vi "Waveforms.vi"(8 "Digital Data":digitaldata={"transitions"=[2, 5, 7, 9, 11, 15], "data"=[[1, 0, 1, 0, 1, 0, 1, 0, 1, 0, 1, 1], [0, 1, 0, 1, 1, 0, 1, 0, 0, 0, 0, 0], [1, 0, 0, 1, 1, 0, 0, 1, 0, 1, 1, 0], [0, 0, 1, 0, 0, 1, 0, 0, 1, 0, 0, 0], [1, 0, 0, 1, 0, 0, 1, 0, 1, 0, 1, 0], [1, 1, 0, 0, 1, 1, 0, 1, 1, 0, 0, 1]]}, 9 "Digital Waveform":digitalwaveform(waveform)={"t0"=timestamp(3352482098.6289887 s since 1904-01-01), "dt"=6.0, "Y"={"transitions"=[3, 4, 7], "data"=[[0, 1, 1, 0, 1, 0, 1], [0, 1, 1, 0, 1, 0, 0], [0, 1, 0, 1, 0, 1, 1]]}}, 10 "Waveform 2":waveform(i64)={"t0"=timestamp(3352482085.4272337 s since 1904-01-01), "dt"=8.0, "Y"=[23, 54, 343]}, 11 "Waveform":waveform(dbl)={"t0"=timestamp(3352482079.508895 s since 1904-01-01), "dt"=3.0, "Y"=[11.0, 22.0, 33.0, 44.0]}) -> (3 "All Default Values Are Equal":bool)   [LabVIEW 2010]
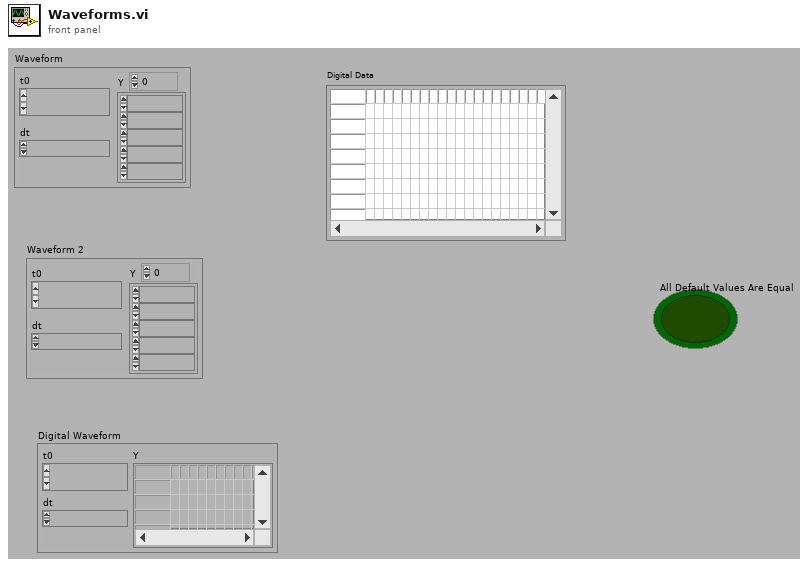
[diagram p1: front panel]
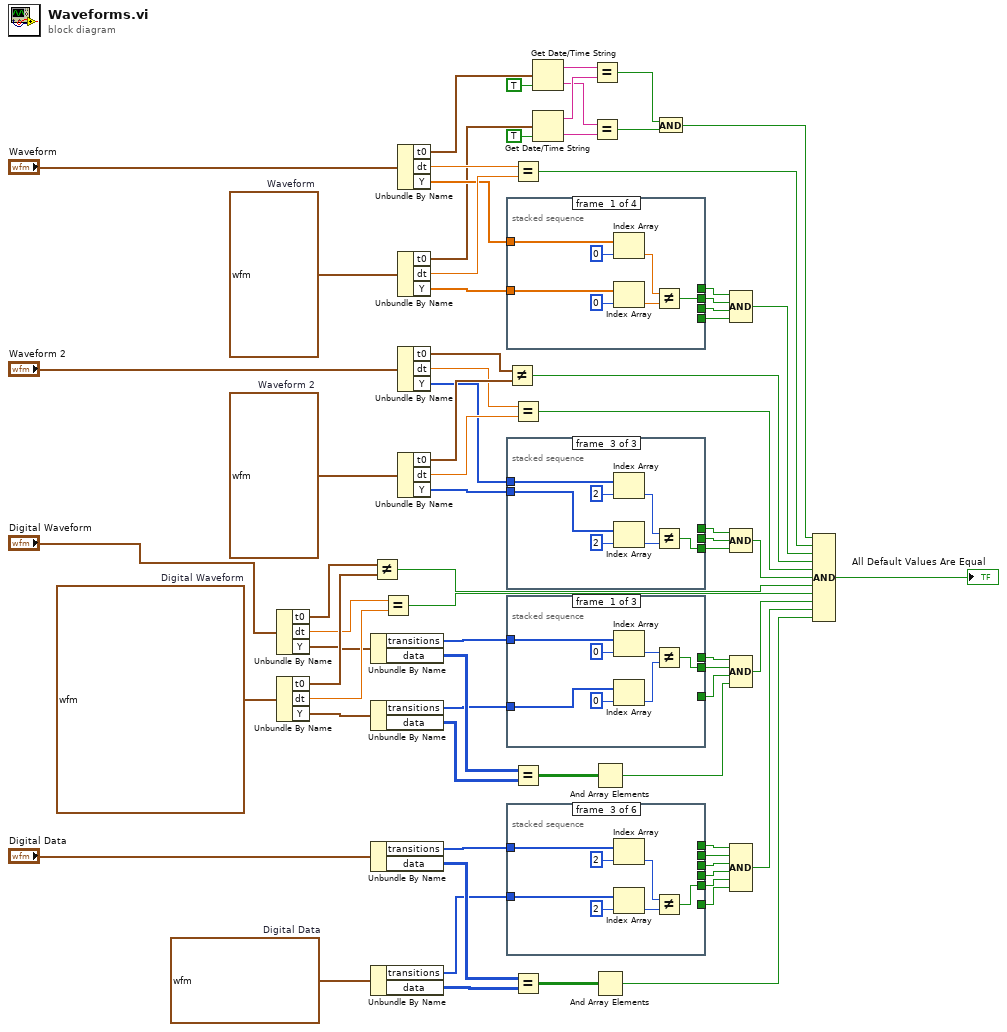
[diagram p0: block diagram]
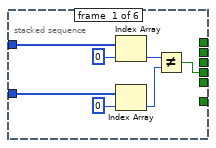
[diagram p2: hidden frame]
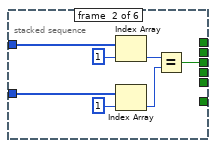
[diagram p3: hidden frame]
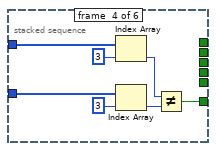
[diagram p4: hidden frame]
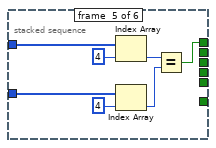
[diagram p5: hidden frame]
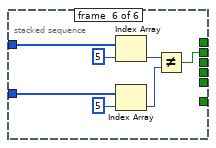
[diagram p6: hidden frame]
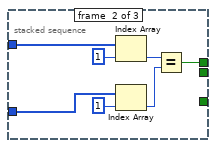
[diagram p7: hidden frame]
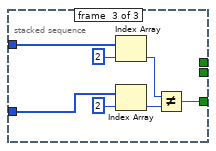
[diagram p8: hidden frame]
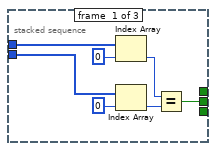
[diagram p9: hidden frame]
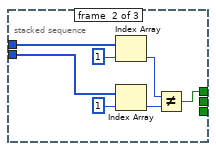
[diagram p10: hidden frame]
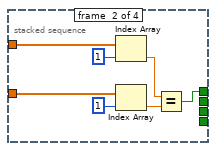
[diagram p11: hidden frame]
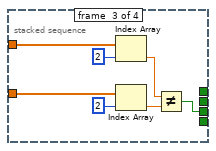
[diagram p12: hidden frame]
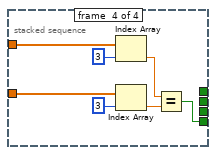
[diagram p13: hidden frame]
diagram:
  w29 = digitaldata {"transitions"=[2, 5, 7, 9, 11, 15], "data"=[[1, 0, 1, 0, 1, 0, 1, 0, 1, 0, 1, 1], [0, 1, 0, 1, 1, 0, 1, 0, 0, 0, 0, 0], [1, 0, 0, 1, 1, 0, 0, 1, 0, 1, 1, 0], [0, 0, 1, 0, 0, 1, 0, 0, 1, 0, 0, 0], [1, 0, 0, 1, 0, 0, 1, 0, 1, 0, 1, 0], [1, 1, 0, 0, 1, 1, 0, 1, 1, 0, 0, 1]]}  # Digital Data
  w39 = digitalwaveform {"t0"=timestamp(3352482098.6289887 s since 1904-01-01), "dt"=6.0, "Y"={"transitions"=[3, 4, 7], "data"=[[0, 1, 1, 0, 1, 0, 1], [0, 1, 1, 0, 1, 0, 0], [0, 1, 0, 1, 0, 1, 1]]}}  # Digital Waveform
  w53 = waveform(i64) {"t0"=timestamp(3352482085.4272337 s since 1904-01-01), "dt"=8.0, "Y"=[23, 54, 343]}  # Waveform 2
  w72 = waveform(dbl) {"t0"=timestamp(3352482079.508895 s since 1904-01-01), "dt"=3.0, "Y"=[11.0, 22.0, 33.0, 44.0]}  # Waveform
  n1 = Unbundle By Name("Digital Waveform") -> ("t0"=w47:timestamp, "dt"=w45:dbl, "Y"=w34:digitaldata)
  n2 = Unbundle By Name(w39) -> ("t0"=w46:timestamp, "dt"=w44:dbl, "Y"=w35:digitaldata)
  n3 = Unbundle By Name(w34) -> ("transitions"=w16:u32[], "data"=w33:u8[][])
  n4 = Unbundle By Name(w35) -> ("transitions"=w15:u32[], "data"=w32:u8[][])
  n5 = Unbundle By Name("Digital Data") -> ("transitions"=w14:u32[], "data"=w21:u8[][])
  n6 = Unbundle By Name(w29) -> ("transitions"=w13:u32[], "data"=w20:u8[][])
  n7 = Not Equal?(x=w47, y=w46) -> (x != y?=w38:bool)
  n8 = Equal?(x=w45, y=w44) -> (x = y?=w37:bool)
  n9 = Unbundle By Name("Waveform") -> ("t0"=w11:timestamp, "dt"=w71:dbl, "Y"=w69:dbl[])
  n10 = Unbundle By Name(w72) -> ("t0"=w10:timestamp, "dt"=w70:dbl, "Y"=w68:dbl[])
  n11 = Unbundle By Name("Waveform 2") -> ("t0"=w63:timestamp, "dt"=w61:dbl, "Y"=w59:i64[])
  n12 = Unbundle By Name(w53) -> ("t0"=w62:timestamp, "dt"=w60:dbl, "Y"=w58:i64[])
  n13 = stacked-sequence {
    tunnel: w69 -> [w80 w87 w94 w101]
    tunnel: w68 -> [w79 w86 w93 w100]
    tunnel: [w74 _ _ _] -> w66
    tunnel: [_ w81 _ _] -> w67
    tunnel: [_ _ w88 _] -> w65
    tunnel: [_ _ _ w95] -> w64
    frame #0 {
      n14 = Index Array(array=w80, index=0) -> (element=w76:dbl)
      n15 = Index Array(array=w79, index=0) -> (element=w75:dbl)
      n16 = Not Equal?(x=w76, y=w75) -> (x != y?=w74:bool)
    }
    frame #1 {
      n17 = Index Array(array=w87, index=1) -> (element=w83:dbl)
      n18 = Index Array(array=w86, index=1) -> (element=w82:dbl)
      n19 = Equal?(x=w83, y=w82) -> (x = y?=w81:bool)
    }
    frame #2 {
      n20 = Index Array(array=w94, index=2) -> (element=w90:dbl)
      n21 = Index Array(array=w93, index=2) -> (element=w89:dbl)
      n22 = Not Equal?(x=w90, y=w89) -> (x != y?=w88:bool)
    }
    frame #3 {
      n23 = Index Array(array=w101, index=3) -> (element=w97:dbl)
      n24 = Index Array(array=w100, index=3) -> (element=w96:dbl)
      n25 = Equal?(x=w97, y=w96) -> (x = y?=w95:bool)
    }
  }
  n26 = Not Equal?(x=w63, y=w62) -> (x != y?=w50:bool)
  n27 = stacked-sequence {
    tunnel: w59 -> [w108 w115 w122]
    tunnel: w58 -> [w107 w114 w121]
    tunnel: [w102 _ _] -> w56
    tunnel: [_ w109 _] -> w57
    tunnel: [_ _ w116] -> w55
    frame #0 {
      n28 = Index Array(array=w108, index=0) -> (element=w104:i64)
      n29 = Index Array(array=w107, index=0) -> (element=w103:i64)
      n30 = Equal?(x=w104, y=w103) -> (x = y?=w102:bool)
    }
    frame #1 {
      n31 = Index Array(array=w115, index=1) -> (element=w111:i64)
      n32 = Index Array(array=w114, index=1) -> (element=w110:i64)
      n33 = Not Equal?(x=w111, y=w110) -> (x != y?=w109:bool)
    }
    frame #2 {
      n34 = Index Array(array=w122, index=2) -> (element=w118:i64)
      n35 = Index Array(array=w121, index=2) -> (element=w117:i64)
      n36 = Not Equal?(x=w118, y=w117) -> (x != y?=w116:bool)
    }
  }
  n37 = stacked-sequence {
    tunnel: w16 -> [w129 w136 w143]
    tunnel: w15 -> [w128 w135 w142]
    tunnel: [w123 _ _] -> w42
    tunnel: [_ w130 _] -> w43
    tunnel: [_ _ w137] -> w41
    frame #0 {
      n38 = Index Array(array=w129, index=0) -> (element=w125:u32)
      n39 = Index Array(array=w128, index=0) -> (element=w124:u32)
      n40 = Not Equal?(x=w125, y=w124) -> (x != y?=w123:bool)
    }
    frame #1 {
      n41 = Index Array(array=w136, index=1) -> (element=w132:u32)
      n42 = Index Array(array=w135, index=1) -> (element=w131:u32)
      n43 = Equal?(x=w132, y=w131) -> (x = y?=w130:bool)
    }
    frame #2 {
      n44 = Index Array(array=w143, index=2) -> (element=w139:u32)
      n45 = Index Array(array=w142, index=2) -> (element=w138:u32)
      n46 = Not Equal?(x=w139, y=w138) -> (x != y?=w137:bool)
    }
  }
  n47 = stacked-sequence {
    tunnel: w14 -> [w150 w157 w164 w171 w178 w185]
    tunnel: w13 -> [w149 w156 w163 w170 w177 w184]
    tunnel: [w144 _ _ _ _ _] -> w25
    tunnel: [_ w151 _ _ _ _] -> w26
    tunnel: [_ _ w158 _ _ _] -> w24
    tunnel: [_ _ _ w165 _ _] -> w23
    tunnel: [_ _ _ _ w172 _] -> w28
    tunnel: [_ _ _ _ _ w179] -> w27
    frame #0 {
      n48 = Index Array(array=w150, index=0) -> (element=w146:u32)
      n49 = Index Array(array=w149, index=0) -> (element=w145:u32)
      n50 = Not Equal?(x=w146, y=w145) -> (x != y?=w144:bool)
    }
    frame #1 {
      n51 = Index Array(array=w157, index=1) -> (element=w153:u32)
      n52 = Index Array(array=w156, index=1) -> (element=w152:u32)
      n53 = Equal?(x=w153, y=w152) -> (x = y?=w151:bool)
    }
    frame #2 {
      n54 = Index Array(array=w164, index=2) -> (element=w160:u32)
      n55 = Index Array(array=w163, index=2) -> (element=w159:u32)
      n56 = Not Equal?(x=w160, y=w159) -> (x != y?=w158:bool)
    }
    frame #3 {
      n57 = Index Array(array=w171, index=3) -> (element=w167:u32)
      n58 = Index Array(array=w170, index=3) -> (element=w166:u32)
      n59 = Not Equal?(x=w167, y=w166) -> (x != y?=w165:bool)
    }
    frame #4 {
      n60 = Index Array(array=w178, index=4) -> (element=w174:u32)
      n61 = Index Array(array=w177, index=4) -> (element=w173:u32)
      n62 = Equal?(x=w174, y=w173) -> (x = y?=w172:bool)
    }
    frame #5 {
      n63 = Index Array(array=w185, index=5) -> (element=w181:u32)
      n64 = Index Array(array=w184, index=5) -> (element=w180:u32)
      n65 = Not Equal?(x=w181, y=w180) -> (x != y?=w179:bool)
    }
  }
  n66 = Equal?(x=w71, y=w70) -> (x = y?=w52:bool)
  n67 = Equal?(x=w61, y=w60) -> (x = y?=w49:bool)
  n68 = Equal?(x=w33, y=w32) -> (x = y?=w31:bool[][])
  n69 = Equal?(x=w21, y=w20) -> (x = y?=w19:bool[][])
  n70 = Get Date/Time String(seconds (now)=w11, want seconds? (F)=TRUE) -> (date string=w4:string, time string=w2:string)  [unwired: 1 in]
  n71 = Get Date/Time String(seconds (now)=w10, want seconds? (F)=TRUE) -> (date string=w3:string, time string=w1:string)  [unwired: 1 in]
  n72 = Equal?(x=w4, y=w3) -> (x = y?=w5:bool)
  n73 = Equal?(x=w2, y=w1) -> (x = y?=w6:bool)
  n74 = And Array Elements(Boolean array=w31) -> (logical AND=w30:bool)
  n75 = And Array Elements(Boolean array=w19) -> (logical AND=w18:bool)
  n76 = And(x=w5, y=w6) -> (x .and. y?=w7:bool)
  n77 = Compound Arithmetic op=AND(w67, w66, w65, w64) -> (w51:bool)
  n78 = Compound Arithmetic op=AND(w57, w56, w55) -> (w48:bool)
  n79 = Compound Arithmetic op=AND(w43, w42, w41, w30) -> (w36:bool)
  n80 = Compound Arithmetic op=AND(w28, w27, w26, w25, w24, w23) -> (w22:bool)
  n81 = Compound Arithmetic op=AND(w7, w52, w51, w50, w49, w48, w38, w37, w36, w22, w18) -> (→"All Default Values Are Equal":bool)
